vi "edtFTPnet.vi"(5 "password":string, 6 "Event":refnum<user-event>, 7 "username":string="anonymous", 8 "错误输入（无错误）":errorcluster, 9 "File List":T1[](array[typedef]), 10 "Port(21)":i32=21, 11 "HostIP":string="127.0.0.1") -> (0 "错误输出":errorcluster, 3 "Success File List":T1[](array[typedef]))   [LabVIEW 2013, in "edtFTPnet.lvlib"]
doc: "---------------------------------------------\n不支持<b>中文</b>命名文件。\n---------------------------------------------"
uses:
  edtFTPnet.lvlib
  Ctrls/edtFTPnet_File.ctl
  Ctrls/edtFTPnet_CallbackEvent.ctl
  Ctrls/edtFTPnet_Action.ctl
  SubVIs/edtFTPnet.dll
panel:
  out "Connected":bool
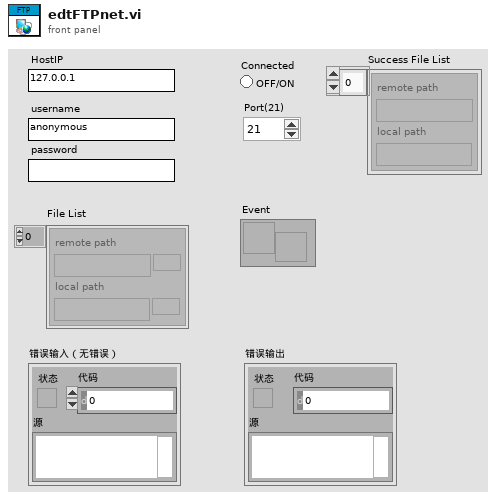
[diagram p1: front panel]
types:
  T1 = typedef "edtFTPnet.lvlib/edtFTPnet_File.ctl" = cluster{"remote path":path, "local path":path}
  T2 = typedef "edtFTPnet.lvlib/edtFTPnet_Session.ctl" = refnum<k24>
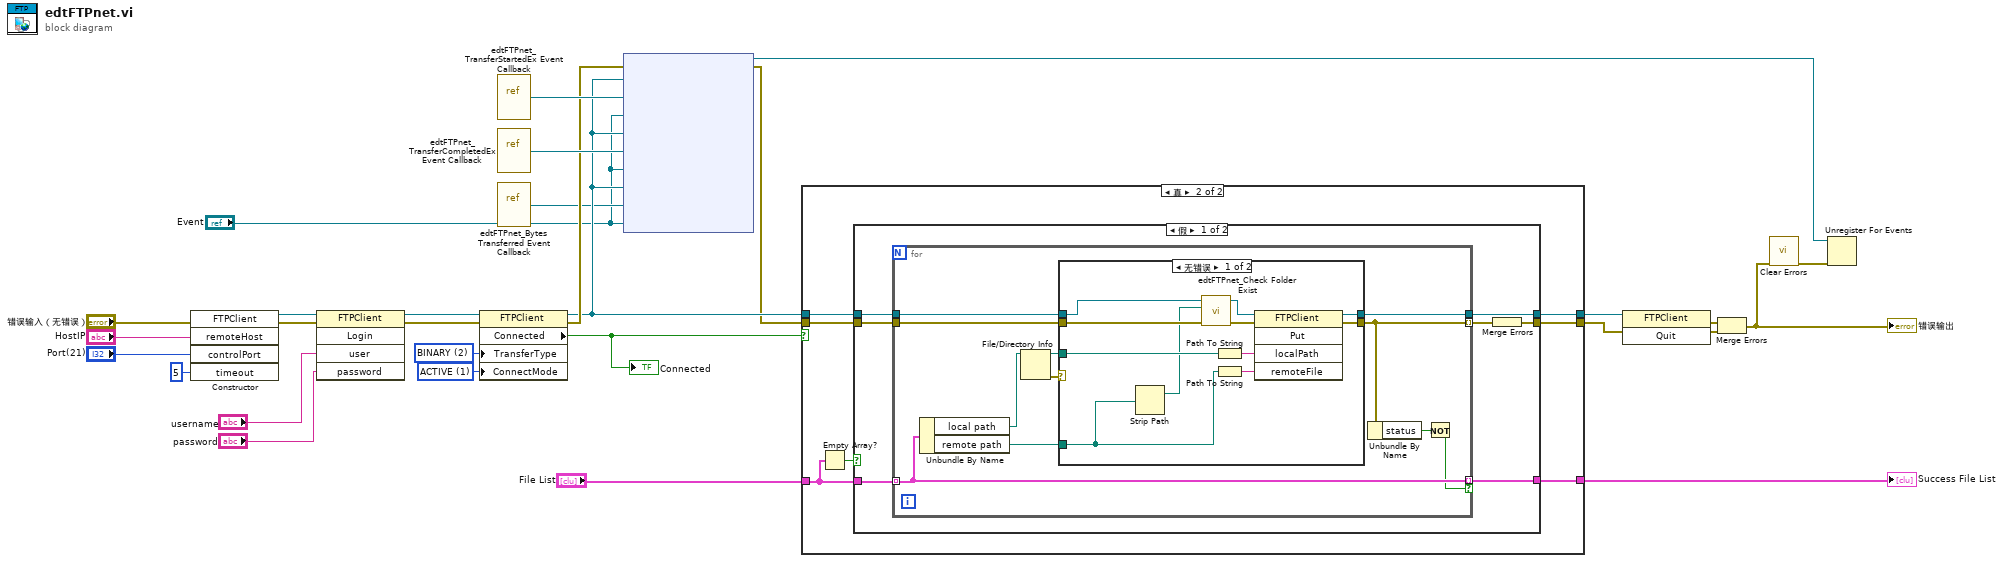
[diagram p0: block diagram]
diagram:
  w14 = 1 items=["ACTIVE"=1, "PASV"=2] ("ConnectMode")
  w15 = 2 items=["ASCII"=1, "BINARY"=2] ("TransferType")
  n1 = constructor class="FTPClient"(error in="错误输入（无错误）", "remoteHost"="HostIP", "controlPort"="Port(21)", "timeout"=5) -> (reference out=w27:refnum<k24>, error out=w12:errorcluster)  [unwired: 2 in, 4 out]
  n2 = invoke class="FTPClient" method="Login"(reference=w27, error in=w12, "user"="username", "password"="password") -> (reference out=w23:refnum<k24>, error out=w24:errorcluster)  [unwired: 1 in, 3 out]
  n3 = property class="FTPClient"(reference=w23, error in=w24, "TransferType"=w15, "ConnectMode"=w14) -> (reference out=w5:refnum<k24>, error out=w9:errorcluster, "Connected"=w16:bool)
  "Connected" <- w16
  n4 = vi-ref "edtFTPnet_TransferStartedEx Event Callback.vi"() -> ("vi reference"=w10:refnum<vi>)
  n5 = vi-ref "edtFTPnet_TransferCompletedEx Event Callback.vi"() -> ("vi reference"=w11:refnum<vi>)
  n6 = vi-ref "edtFTPnet_Bytes Transferred Event Callback.vi"() -> ("vi reference"=w4:refnum<vi>)
  n7 = node(w9, w5, w10, "Event", w5, w11, "Event", w5, w4, "Event") -> (w8:refnum<k27>, w3:errorcluster)  [unwired: 1 in]
  n8 = case shown="真" w16 {
    tunnel: w3 -> [w29 w31]
    tunnel: [w30 w36] -> w19
    tunnel: [w29 w35] -> w13
    tunnel: "File List" -> [_ w34]
    tunnel: w5 -> [w30 w32]
    tunnel: [_ w33] -> w1
    frame False {
    }
    frame True {
      n9 = Empty Array?(array=w34) -> (empty?=w37:bool)
      n10 = case shown="假" w37 {
        tunnel: w31 -> [w44 w69]
        tunnel: w32 -> [w43 w70]
        tunnel: [w40 w69] -> w35
        tunnel: w34 -> [w39 _]
        tunnel: [w41 w70] -> w36
        tunnel: [w38 _] -> w33
        frame False {
          n11 = for {
            tunnel: w44 -> [w55]
            tunnel: w43 -> [w54]
            tunnel: [w48] -> w42 mode=indexing
            tunnel: [w49] -> w41
            tunnel: w39 -> [w47] mode=indexing
            tunnel: [w47] -> w38 mode=indexing if=w45
            n12 = Unbundle By Name(w47) -> ("local path"=w52:path, "remote path"=w53:path)
            n13 = File/Directory Info(path=w52) -> (path out=w50:path, error out=w51:errorcluster)  [unwired: 1 in, 5 out]
            n14 = case shown="无错误" w51 {
              tunnel: [w65 w68] -> w48
              tunnel: w55 -> [w60 w68]
              tunnel: w54 -> [w62 w67]
              tunnel: [w66 w67] -> w49
              tunnel: w53 -> [w57 _]
              tunnel: w50 -> [w58 _]
              frame No Error {
                n15 = Strip Path(path=w57) -> (stripped path=w56:path)  [unwired: 1 out]
                n16 = call "edtFTPnet_Check Folder Exist.vi"("error in(no error)"=w60, "remote folder path"=w56, "FTPClient in"=w62) -> ("error out"=w59:errorcluster, "FTPClient out"=w61:T2)  [unwired: 7 in]
                n17 = Path To String(path=w58) -> (string=w64:string)
                n18 = Path To String(path=w57) -> (string=w63:string)
                n19 = invoke class="FTPClient" method="Put"(reference=w61, error in=w59, "localPath"=w64, "remoteFile"=w63) -> (reference out=w66:T2, error out=w65:errorcluster)  [unwired: 1 in, 3 out]
              }
              frame Error {
              }
            }
            n20 = Unbundle By Name(w48) -> ("status"=w46:bool)
            n21 = Not(x=w46) -> (.not. x?=w45:bool)
          }
          n22 = Merge Errors(w42) -> (w40:errorcluster)
        }
        frame True {
        }
      }
    }
  }
  "Success File List" <- w1
  n23 = invoke class="FTPClient" method="Quit"(reference=w19) -> (error out=w18:errorcluster)  [unwired: 2 in, 2 out]
  n24 = Merge Errors(w18, w13) -> (w7:errorcluster)
  "错误输出" <- w7
  n25 = call <vilib>:"Clear Errors.vi"("error in (no error)"=w7) -> ("error out"=w6:errorcluster)  [unwired: 6 in]
  n26 = Unregister For Events(event registration refnum=w8, error in=w6) -> ()  [unwired: 1 out]
